vi "Launcher.vi"   [LabVIEW 2020]
uses:
  Caller/Caller/Caller.lvclass
  C:/Program Files/National Instruments/LabVIEW 2020/vi.lib/ActorFramework/Actor/Actor.lvclass
  Nested/Nested/Nested.lvclass
  <vilib>/ActorFramework/Actor/Actor.lvclass
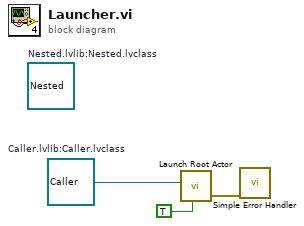
[diagram p0: block diagram]
diagram:
  (unwired) refnum<class "Nested.lvclass"> refnum  # Nested.lvlib:Nested.lvclass
  w1 = refnum<class "Caller.lvclass"> refnum  # Caller.lvlib:Caller.lvclass
  n1 = call <vilib>:"Launch Root Actor.vi"("Open Actor Core front panel? (F)"=TRUE, "Actor"=w1) -> ("error out"=w2:errorcluster)  [unwired: 8 in, 1 out]
  n2 = call <vilib>:"Simple Error Handler.vi"("error in (no error)"=w2) -> ()  [unwired: 4 in, 5 out]
